vi "WPI_CameraNotifier GUID.vi"() -> (3 "Notifier GUID":string="{58B0A275-1E2D-480c-9B20-695A385A3C3F}")   [LabVIEW 2017]
doc: "This software is licensed. Open the labview\\readme\\WPI Robotics Library Open Source License.txt file for more information."
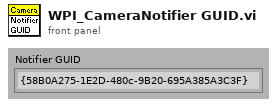
[diagram p1: front panel]
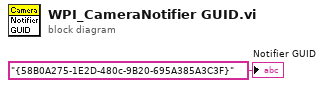
[diagram p0: block diagram]
diagram:
  "Notifier GUID" <- "{58B0A275-1E2D-480c-9B20-695A385A3C3F}"
